vi "NMEA serial.vi"() -> ()   [LabVIEW 2016, in "环境动力监测库.lvlib" / "AIRMAR WeatherCaster.lvlib"]
uses:
  AIRMAR WeatherCaster.lvlib
  NMEA_WIMDA-data.ctl
  NMEA_GPRMC-data.ctl
  NMEA_LatitudeDirection.ctl
  NMEA_LongitudeDirection.ctl
  <vilib>/Utility/miscctls.llb/LVPointTypeDef.ctl
  <vilib>/Instr/_visa.llb/VISA Configure Serial Port (Instr).vi
  <vilib>/ptbypt/NI_PtbyPt.lvlib
  <vilib>/Utility/config.llb/NI_LVConfig.lvlib
panel:
  out "气温":dbl
  out "气压":dbl
  out "风速":dbl
  out "风向":dbl
  out "偏移量/米":dbl format="%#.2f"
  out "纬度":dbl
  out "经度":dbl
  out "时间":timestamp format="%<%H:%M:%S>T"
  out "日期":timestamp format="%<%Y/%m/%d>T"
  out "浮标投放点":cluster{"纬度":dbl, "经度":dbl}
  out "波特率":u32
  out "串口":string
  out "WIMDA signal":bool=TRUE
  in  "重新定标":bool
  in  "移位报警设定值":u32=1000
  out "$GPRMC-message_OUT":T1={"TimeStamp"=timestamp(0 s since 1904-01-01), "Validity"=FALSE, "Latitude"=0.0, "Latitude-Direction"=enum."North", "Longitude"=0.0, "Longitude-Direction"=enum."East", "Speed in knots"=0.0, "True course"=0.0, "Date Stamp"=timestamp(0 s since 1904-01-01), "Magnetic Variation (East/West)"=0.0} {"Magnetic Variation (East/West)" format="%.02f [deg]"; "Date Stamp" format="%<%x>T"; "True course" format="%.02f [deg]"; "Speed in knots" format="%.02f [kts]"; "Longitude" format="%0.4f [long]"; "Latitude" format="%.04f [lat]"; "TimeStamp" format="%<%.2X>T"}
  out "匹配语句":string
  out "$WIMDA-message_OUT":T4
  in  "串口打开":bool
  out "RAW DATA":string
  in  "baud rate (9600)":u32(ring)=4800 caption="波特率" items=["1200"=1200, "2400"=2400, "4800"=4800, "9600"=9600, "38400"=38400, "115200"=115200]
  in  "VISA resource name":refnum<visa-resource-name> caption="串口"
  # "℃"
  # "bars"
  # "m/s"
  # "米"
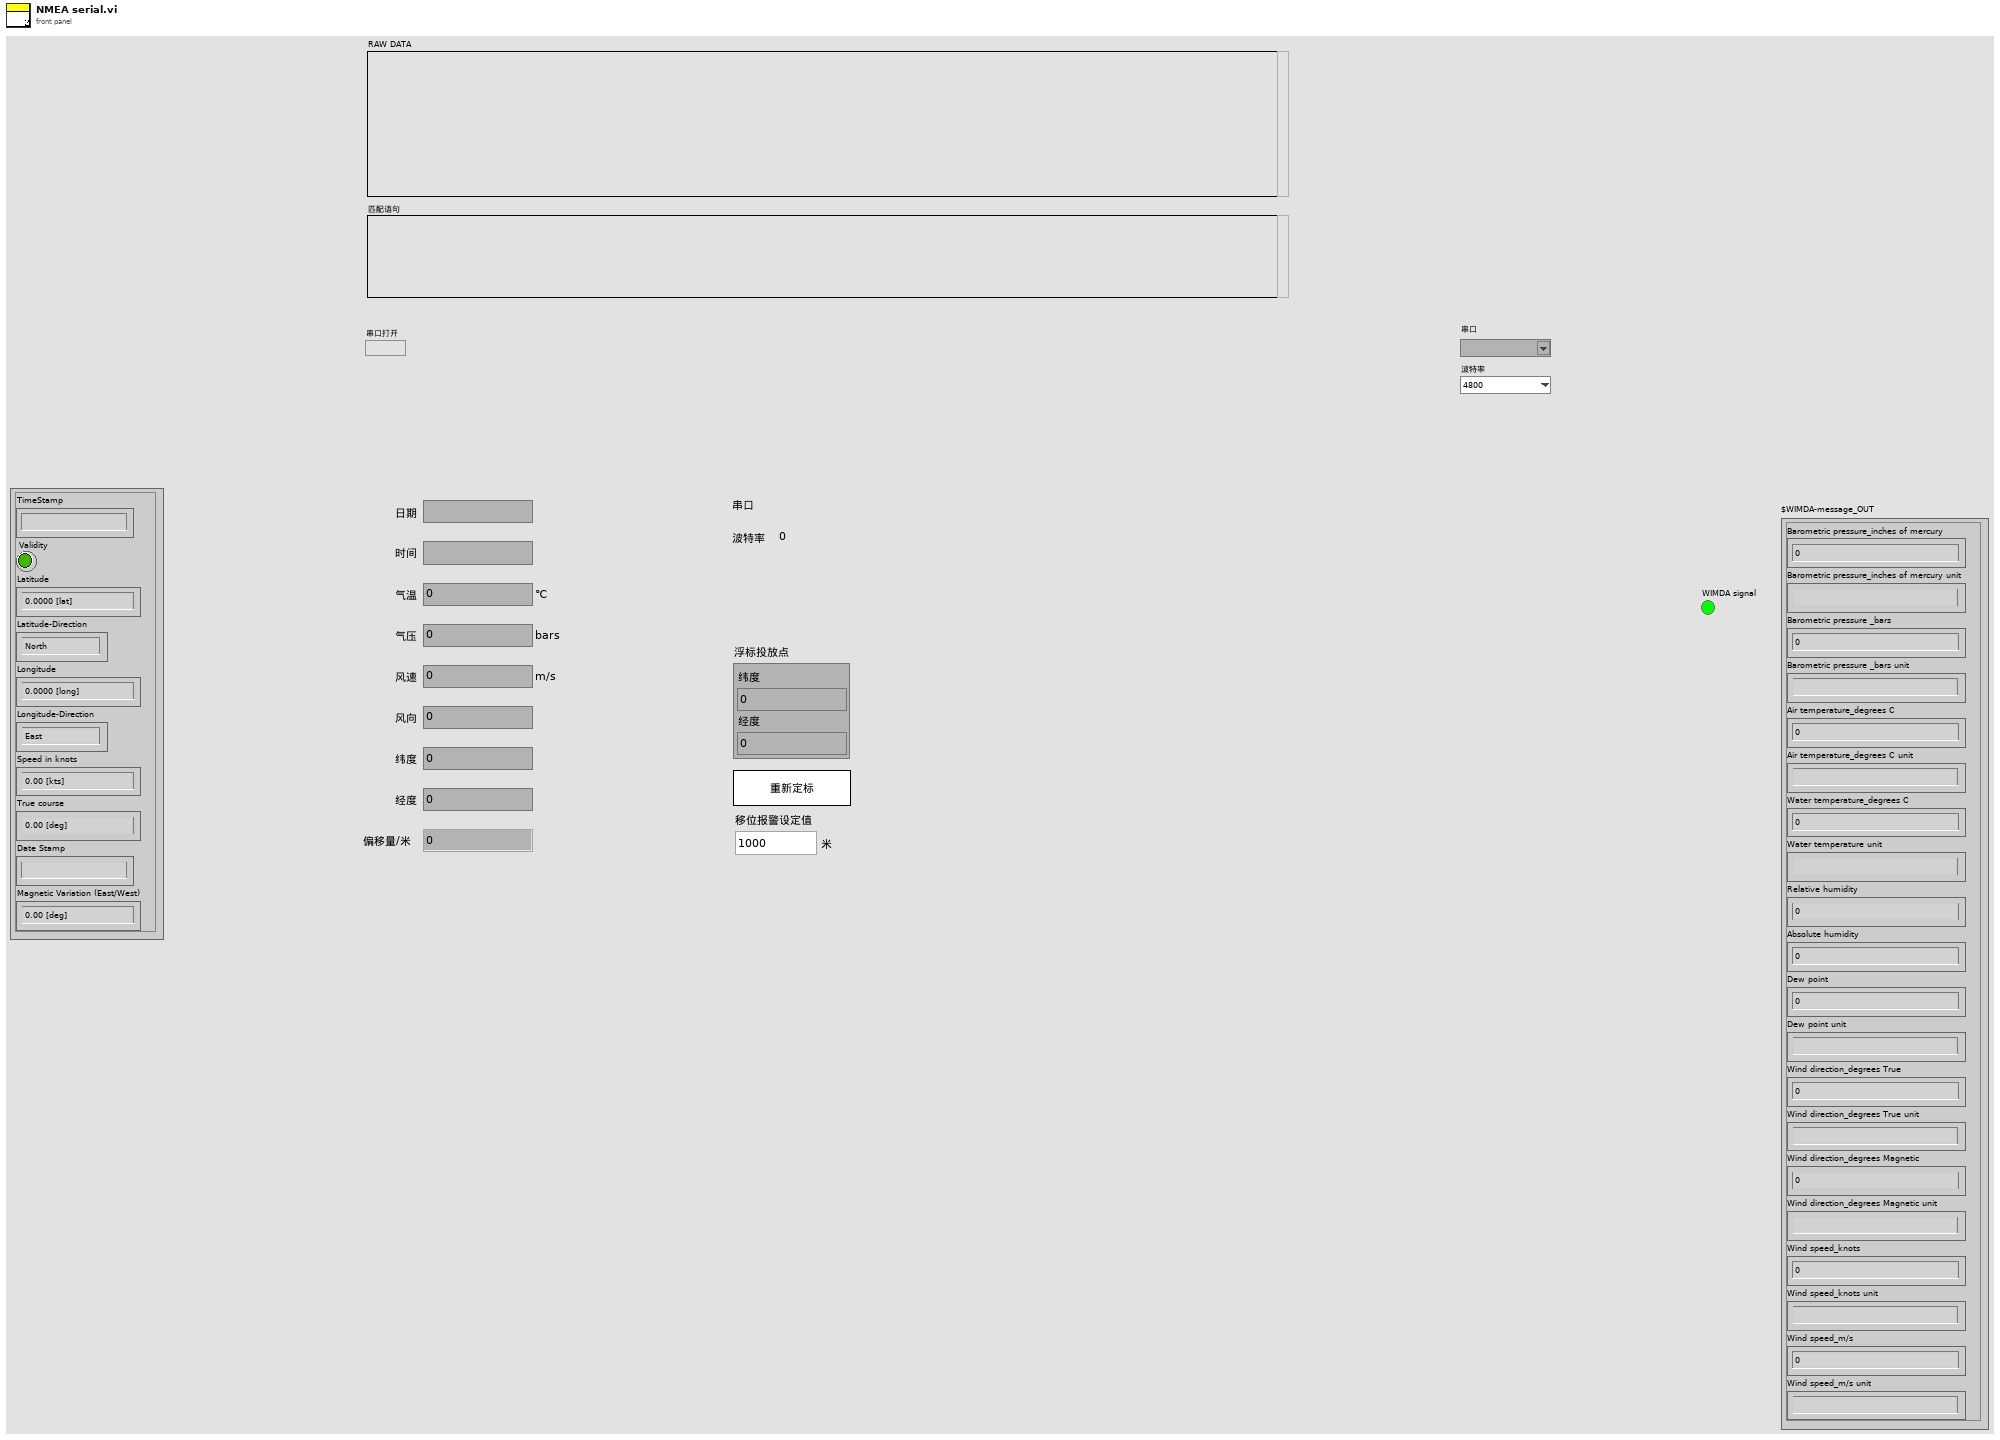
[diagram p1: front panel]
types:
  T1 = typedef "环境动力监测库.lvlib/AIRMAR WeatherCaster.lvlib/NMEA_GPRMC-data.ctl" = cluster{"TimeStamp":timestamp, "Validity":bool, "Latitude":dbl, "Latitude-Direction":T2, "Longitude":dbl, "Longitude-Direction":T3, "Speed in knots":dbl, "True course":dbl, "Date Stamp":timestamp, "Magnetic Variation (East/West)":dbl}
  T2 = typedef "环境动力监测库.lvlib/AIRMAR WeatherCaster.lvlib/NMEA_LatitudeDirection.ctl" = enum16{"", "North", "South"}
  T3 = typedef "环境动力监测库.lvlib/AIRMAR WeatherCaster.lvlib/NMEA_LongitudeDirection.ctl" = enum16{"", "East", "West"}
  T4 = typedef "环境动力监测库.lvlib/AIRMAR WeatherCaster.lvlib/NMEA_WIMDA-data.ctl" = cluster{"Barometric pressure_inches of mercury":dbl, "Barometric pressure_inches of mercury unit":string, "Barometric pressure _bars":dbl, "Barometric pressure _bars unit":string, "Air temperature_degrees C":dbl, "Air temperature_degrees C unit":string, "Water temperature_degrees C":dbl, "Water temperature unit":string, "Relative humidity":dbl, "Absolute humidity":dbl, "Dew point":dbl, "Dew point unit":string, "Wind direction_degrees True":dbl, "Wind direction_degrees True unit":string, "Wind direction_degrees Magnetic":dbl, "Wind direction_degrees Magnetic unit":string, "Wind speed_knots":dbl, "Wind speed_knots unit":string, "Wind speed_m/s":dbl, "Wind speed_m/s unit":string}
  T5 = typedef "LVPointTypeDef.ctl" = cluster{"Horizontal":i16, "Vertical":i16}
  T6 = typedef "LVDateTimeRec.ctl" = cluster{"秒数的小数部分":dbl, "秒":i32, "分":i32, "时":i32, "日":i32, "月":i32, "年":i32, "天数（周）":i32, "天数（年）":i32, "DST":i32}
  T7 = cluster{"漏水监测输出":cluster{"漏水监测告警":bool, "告警内容":string}, "门禁监测输出":cluster{"门禁监测告警":bool, "告警内容":string}, "门禁监测输出2":cluster{"门禁监测告警":bool, "告警内容":string}, "温湿度监测输出":cluster{"温湿度监测告警":bool, "告警内容":string}, "烟雾监测输出":cluster{"烟雾监测告警":bool, "告警内容":string}, "空调监测输出":cluster{"空调监测告警":bool, "告警内容":string}, "自动重合闸输出":cluster{"自动重合闸告警":bool, "告警内容":string}, "红外入侵输出":cluster{"红外入侵告警":bool, "告警内容":string}, "振动输出":cluster{"振动告警":bool, "告警内容":string}, "UPS输出":cluster{"UPS告警":bool, "告警内容":string}, "蓄电池输出":cluster{"蓄电池告警":bool, "告警内容":string}, "蓄电池输出2":cluster{"蓄电池告警":bool, "告警内容":string}, "GPS输出":cluster{"定位告警":bool, "告警内容":string}, "北斗输出":cluster{"定位告警":bool, "告警内容":string}, "气象输出":cluster{"气象告警":bool, "告警内容":string}, "废液输出":cluster{"废液告警":bool, "告警内容":string}, "废液输出2":cluster{"废液告警":bool, "告警内容":string}}
  T8 = cluster{"监测项描述:输出":string, "连接方式":enum16{"串口", "TCP"}, "端口":string, "IP address:":string, "Port:":string, "站号":u64, "传感器型号":string, "波特率":u64, "data bits":u64, "停止位":u16, "奇偶校验":u16}
  T9 = typedef "NI_LVConfig.lvlib/Config Data RefNum.ctl" = refnum<k1>
  T10 = enum8{"Enabled", "Disabled", "Disabled and Grayed Out"}
  T11 = cluster{"传感器":cluster{"红外监测":cluster{"红外监测":bool, "红外入侵监测":bool}, "振动监测":cluster{"振动监测":bool, "振动监测 2":bool}, "烟雾监测":cluster{"烟雾监测":bool, "烟雾监测 2":bool}, "门禁监测":cluster{"门禁监测":bool, "门禁开关监测":bool}, "门禁2监测":cluster{"门禁监测2":bool, "门禁开关监测2":bool}, "水浸监测":cluster{"水浸监测":bool, "漏水详情":bool}, "废液监测":cluster{"废液监测":bool, "废液详情":bool}, "废液监测2":cluster{"废液监测2":bool, "废液2详情":bool}}, "气象仪":cluster{"气温: ":sgl, "气压: ":sgl, "风速:":sgl, "风向:":sgl, "气象仪经度: ":sgl, "气象仪纬度: ":sgl, "详情  ":bool}}
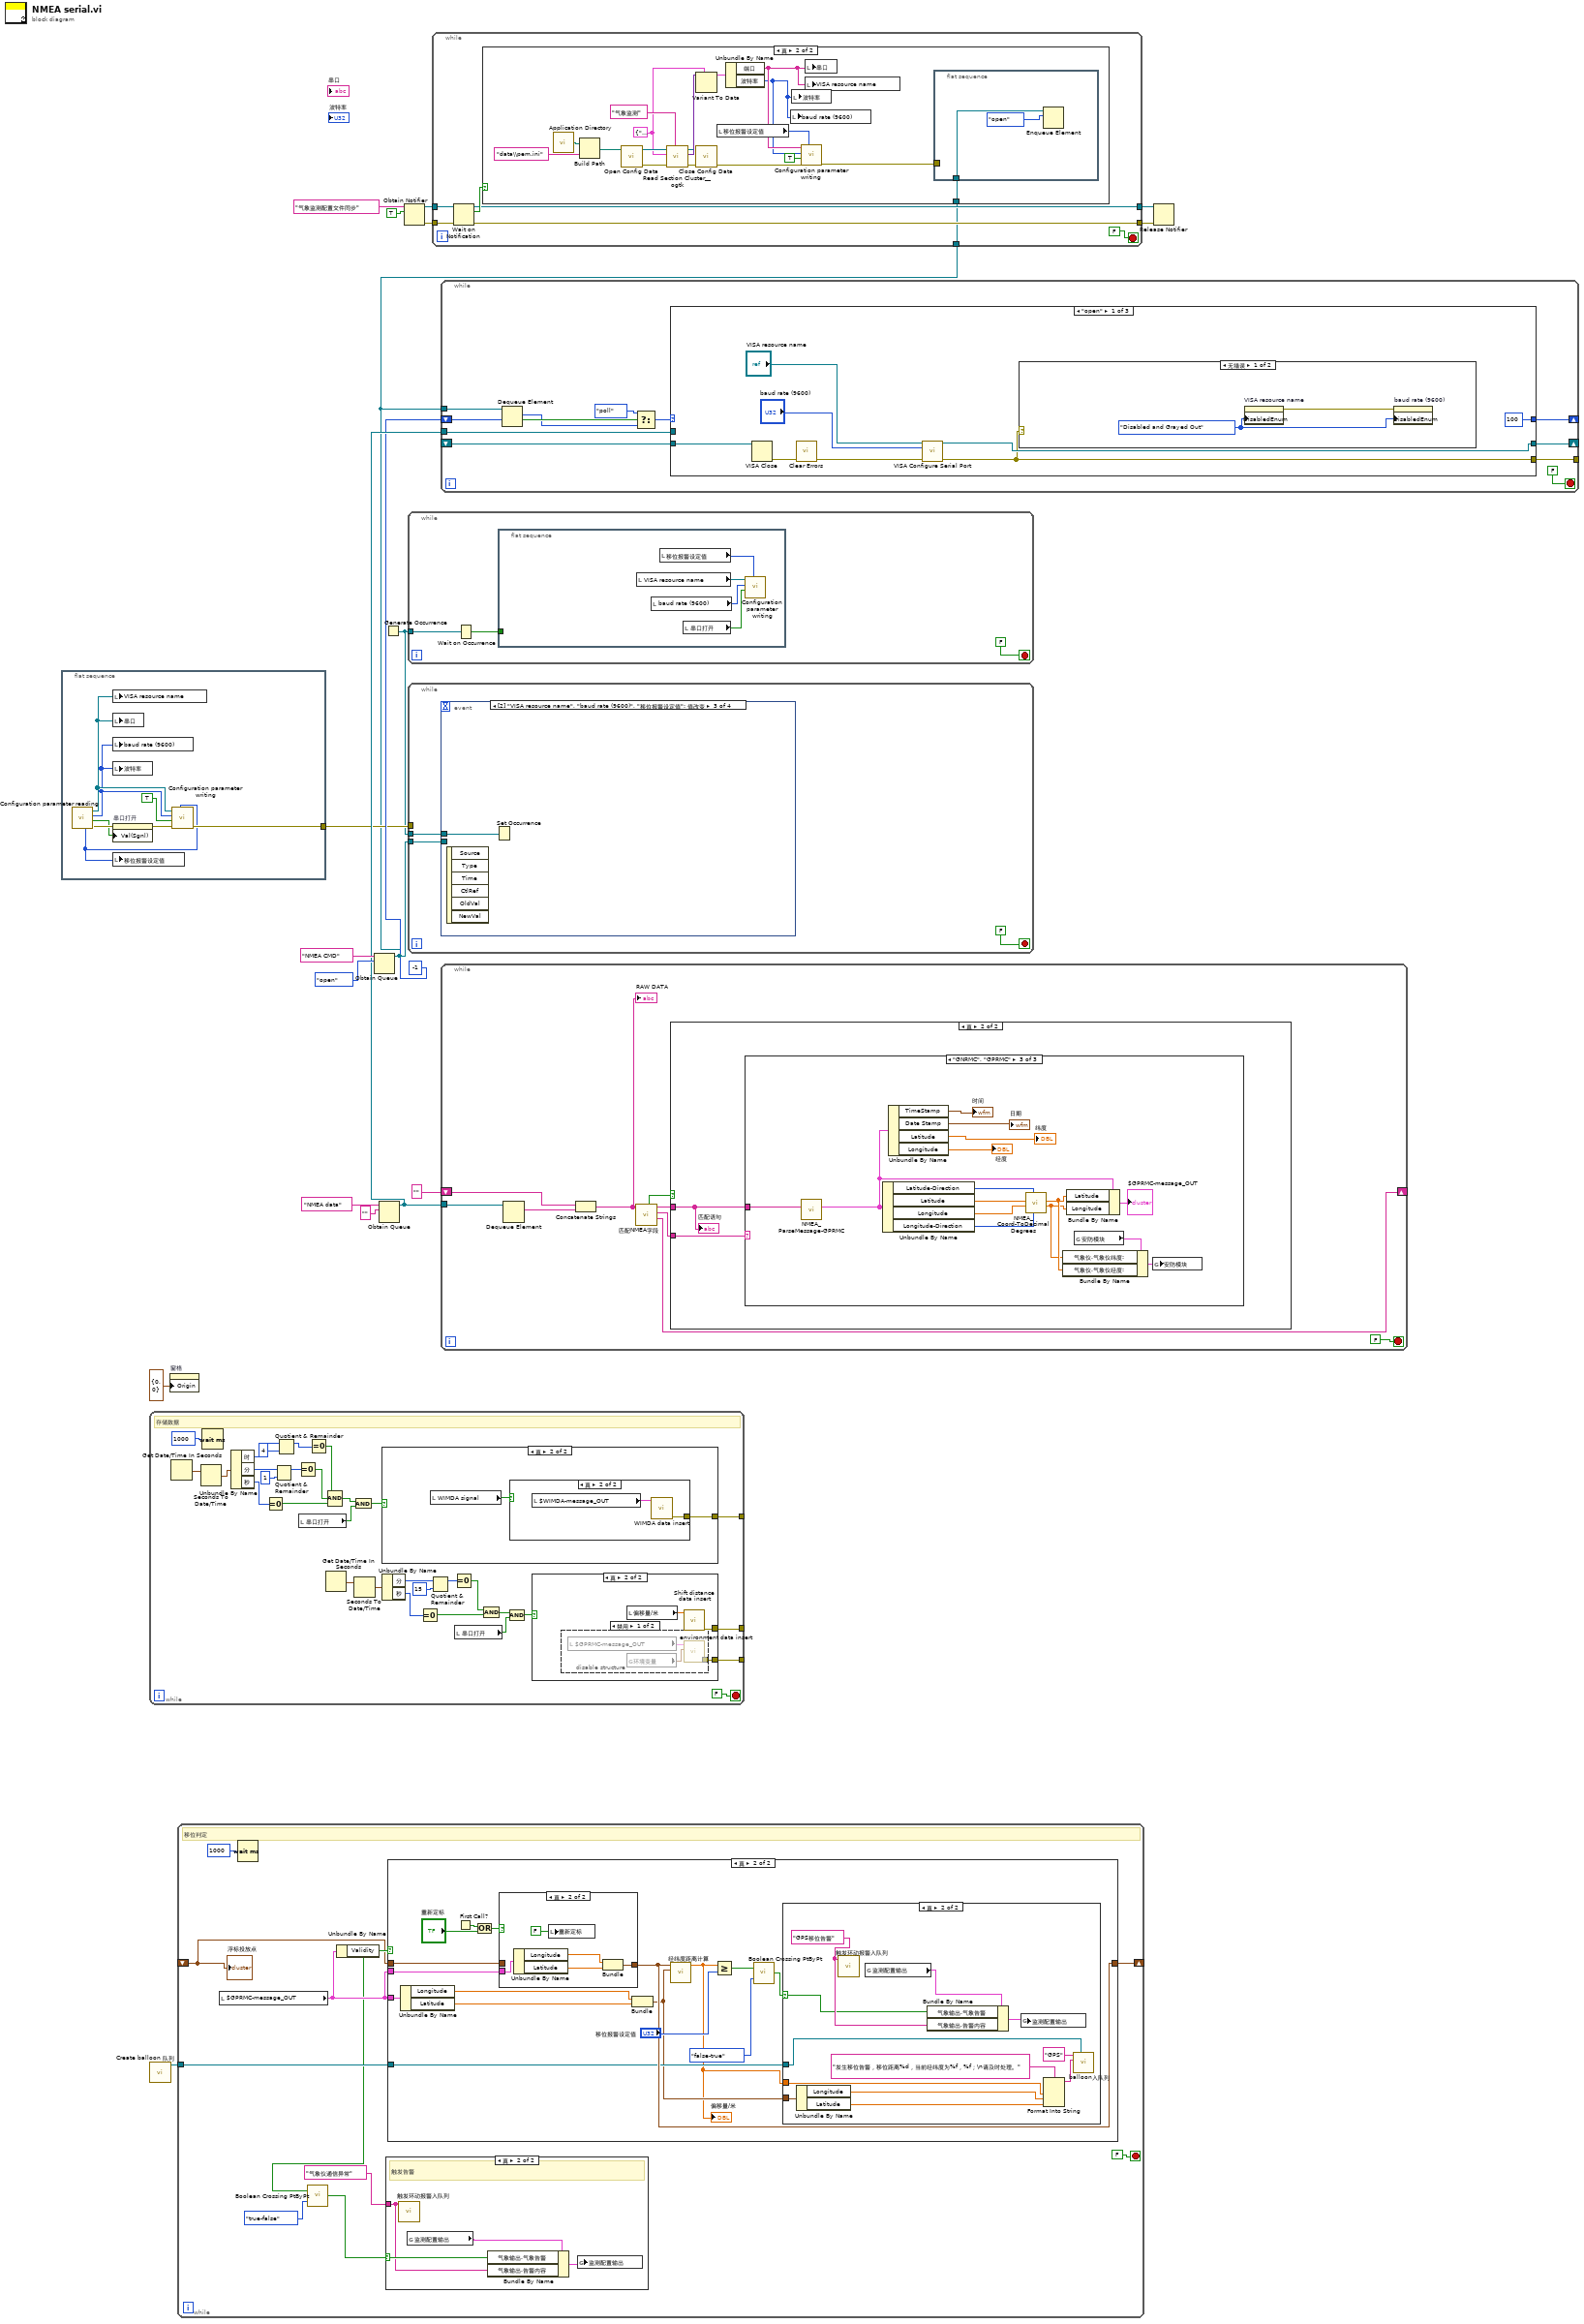
[diagram p0: block diagram]
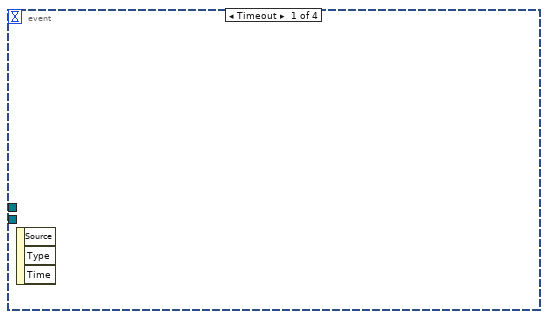
[diagram p11: hidden frame]
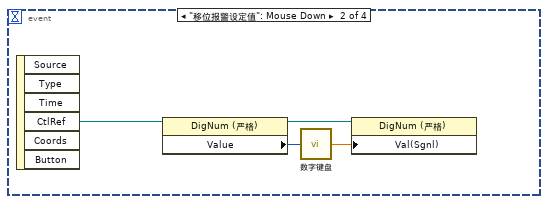
[diagram p12: hidden frame]
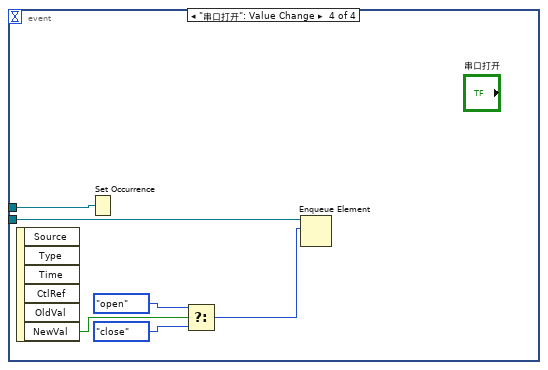
[diagram p13: hidden frame]
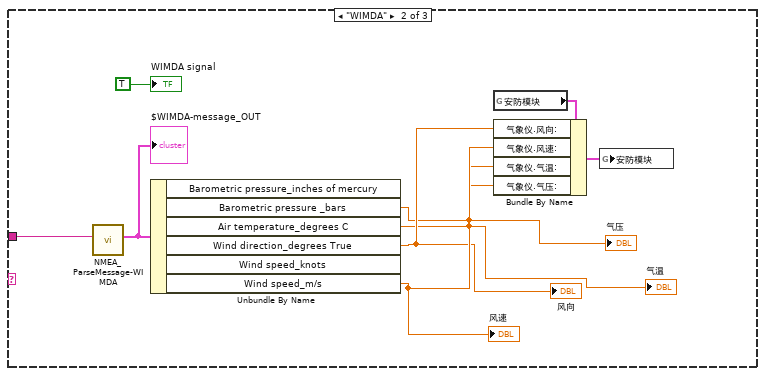
[diagram p16: hidden frame]
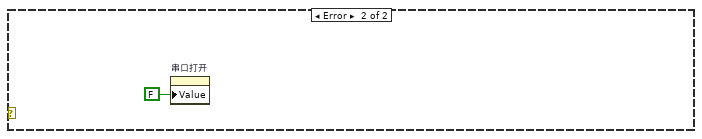
[diagram p17: hidden frame]
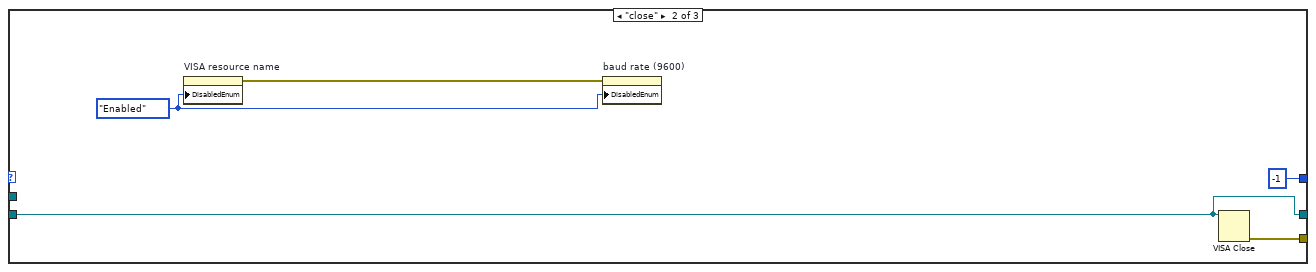
[diagram p18: hidden frame]
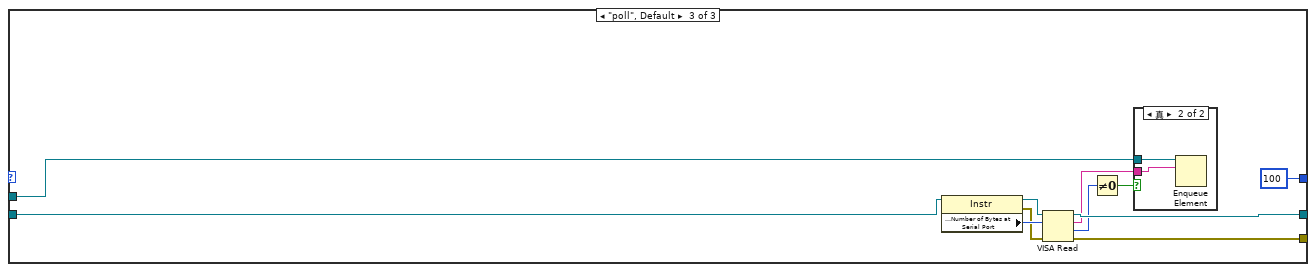
[diagram p19: hidden frame]
diagram:
  n1 = flat-sequence {
    tunnel: [w20] -> w10
    frame #0 {
      n2 = call "Configuration parameter reading.vi"() -> ("error out"=w26:errorcluster, "enable"=w25:bool, "baud rate (9600)"=w23:u32, "VISA resource name"=w24:refnum<visa-resource-name>, "Shift distance"=w19:u32)  [unwired: 7 in]
      n3 = local write "VISA resource name"(w24) -> ()
      n4 = local write "串口"(w24) -> ()
      n5 = local write "baud rate (9600)"(w23) -> ()
      n6 = local write "波特率"(w23) -> ()
      n7 = property on="串口打开" class="Bool (严格)"(error in=w26, "Val(Sgnl)"=w25) -> (error out=w21:errorcluster)  [unwired: 1 in, 1 out]
      n8 = local write "移位报警设定值"(w19) -> ()
      n9 = call "Configuration parameter writing.vi"("Shift distance"=w19, "error in (no error)"=w21, "enable"=TRUE, "baud rate (9600)"=w23, "VISA resource name"=w24) -> ("error out"=w20:errorcluster)  [unwired: 6 in]
    }
  }
  n10 = while {
    tunnel: [w35] -> _
    tunnel: [w34] -> _
    tunnel: [w33] -> _
    stop <- FALSE stop-if-true
    # "存储数据"
    n11 = Get Date/Time In Seconds() -> (seconds since 1Jan1904=w48:timestamp)
    n12 = Seconds To Date/Time(time stamp (now)=w48) -> (date time rec=w56:T6)  [unwired: 1 in]
    n13 = Wait (ms)(milliseconds to wait=u32 1000 ("等待时间（毫秒）")) -> ()  [unwired: 1 out]
    n14 = Unbundle By Name(w56) -> ("时"=w30:i32, "分"=w55:i32, "秒"=w52:i32)
    n15 = Equal To 0?(x=w52) -> (x = 0?=w50:bool)
    n16 = Quotient & Remainder(x=w55, y=1) -> (x-y*floor(x/y)=w53:i32)  [unwired: 1 out]
    n17 = Quotient & Remainder(x=w30, y=4) -> (x-y*floor(x/y)=w28:i32)  [unwired: 1 out]
    n18 = Equal To 0?(x=w53) -> (x = 0?=w51:bool)
    n19 = local read "串口打开"() -> (w45:bool)
    n20 = Equal To 0?(x=w28) -> (x = 0?=w27:bool)
    n21 = Get Date/Time In Seconds() -> (seconds since 1Jan1904=w44:timestamp)
    n22 = Compound Arithmetic op=AND ("复合运算")(w27, w51, w50) -> (w49:bool)
    n23 = And(x=w49, y=w45) -> (x .and. y?=w46:bool)
    n24 = Seconds To Date/Time(time stamp (now)=w44) -> (date time rec=w37:T6)  [unwired: 1 in]
    n25 = case shown="真" w46 {
      tunnel: [_ w65] -> w34
      frame False {
      }
      frame True {
        n26 = local read "WIMDA signal"() -> (w64:bool)
        n27 = case shown="真" w64 {
          tunnel: [_ w66] -> w65
          frame False {
          }
          frame True {
            n28 = local read "$WIMDA-message_OUT"() -> (w67:T4)
            n29 = call "WIMDA data insert.vi"("WIMDA-data"=w67) -> ("error out"=w66:errorcluster)  [unwired: 10 in]
          }
        }
      }
    }
    n30 = Unbundle By Name(w37) -> ("分"=w38:i32, "秒"=w41:i32)
    n31 = Equal To 0?(x=w41) -> (x = 0?=w43:bool)
    n32 = Quotient & Remainder(x=w38, y=15) -> (x-y*floor(x/y)=w40:i32)  [unwired: 1 out]
    n33 = Equal To 0?(x=w40) -> (x = 0?=w42:bool)
    n34 = local read "串口打开"() -> (w32:bool)
    n35 = And(x=w42, y=w43) -> (x .and. y?=w31:bool)
    n36 = Compound Arithmetic op=AND ("复合运算")(w31, w32) -> (w36:bool)
    n37 = case shown="真" w36 {
      tunnel: [_ w60] -> w35
      tunnel: [_ w59] -> w33
      frame False {
      }
      frame True {
        n38 = disable-structure shown="禁用" {
          disable-tunnel: [w63 _] -> w60
          frame Disabled {
            n39 = local read "$GPRMC-message_OUT"() -> (w62:T1)
            n40 = global read "气象全局变量.vi" "环境变量"() -> (w61:cluster{"电压":dbl, "室温":dbl, "湿度":dbl})
            n41 = call "environment data insert.vi"("环境变量"=w61, "$GPRMC-message_OUT"=w62) -> ("error out"=w63:errorcluster)  [unwired: 9 in]
          }
          frame Enabled {
          }
        }
        n42 = local read "偏移量/米"() -> (w58:dbl)
        n43 = call "Shift distance data insert.vi"("移位距离"=w58) -> ("error out"=w59:errorcluster)  [unwired: 10 in]
      }
    }
  }
  n44 = call "Create balloon 队列.vi"() -> ("队列输出"=w8:refnum<queue>)  [unwired: 11 in]
  n45 = property on="窗格" class="Pane"("Origin"=T5 {"Horizontal"=0, "Vertical"=0} ("原点")) -> ()  [unwired: 2 in, 2 out]
  n46 = while {
    shift-right: [w77] -> _
    shift-left: _ -> [w68]
    tunnel: w8 -> [w73]
    stop <- FALSE stop-if-true
    # "移位判定"
    n47 = local read "$GPRMC-message_OUT"() -> (w75:T1)
    n48 = Wait (ms)(milliseconds to wait=u32 1000 ("等待时间（毫秒）")) -> ()  [unwired: 1 out]
    n49 = Unbundle By Name(w75) -> ("Validity"=w69:bool)
    n50 = call <vilib>:"Boolean Crossing PtByPt.vi"("direction"=enum16{"either", "false-true", "true-false"}."true-false", "input"=w69) -> ("crossing"=w71:bool)  [unwired: 1 in]
    n51 = case shown="真" w71 {
      selector: w71 -> [_ w81]
      tunnel: "气象仪通信异常" ("设备") -> [_ w80]
      frame False {
      }
      frame True {
        # "触发告警"
        n52 = call "触发环动报警入队列.vi"("报警内容"=w80) -> ()  [unwired: 11 in]
        n53 = global read "内部交互全局变量.vi" "监测配置输出"() -> (w79:T7)
        n54 = Bundle By Name(cluster=w79, "气象输出.气象告警"=w81, "气象输出.告警内容"=w80) -> (w78:T7)
        n55 = global write "内部交互全局变量.vi" "监测配置输出"(w78) -> ()
      }
    }
    n56 = case shown="真" w69 {
      tunnel: [w82 w96] -> w77
      tunnel: w68 -> [w82 w95]
      tunnel: w75 -> [_ w94]
      tunnel: w75 -> [_ w93]
      tunnel: w73 -> [_ w89]
      frame False {
      }
      frame True {
        n57 = Unbundle By Name(w93) -> ("Longitude"=w98:dbl, "Latitude"=w97:dbl)
        n58 = First Call?() -> (First Call?: T/F=w92:bool)
        n59 = Or(x=w92, y="重新定标") -> (x .or. y?=w91:bool)
        n60 = case shown="真" w91 {
          tunnel: [w111 w114] -> w96
          tunnel: w95 -> [w111 _]
          tunnel: w94 -> [_ w113]
          frame False {
          }
          frame True {
            n61 = Unbundle By Name(w113) -> ("Longitude"=w115:dbl, "Latitude"=w116:dbl)
            n62 = local write "重新定标"(FALSE ("重新定标")) -> ()
            n63 = Bundle("Longitude"=w115, "Latitude"=w116) -> (w114:cluster{"Longitude":dbl, "Latitude":dbl})  [unwired: 1 in]
          }
        }
        n64 = Bundle("Longitude"=w98, "Latitude"=w97) -> (w84:cluster{"Longitude":dbl, "Latitude":dbl})  [unwired: 1 in]
        n65 = call "经纬度距离计算.vi"("结束位置"=w84, "起始位置"=w96) -> ("距离"=w83:dbl)  [unwired: 9 in]
        "偏移量/米" <- w83
        n66 = Greater Or Equal?(x=w83, y="移位报警设定值") -> (x >= y?=w87:bool)
        n67 = call <vilib>:"Boolean Crossing PtByPt.vi"("direction"=enum16{"either", "false-true", "true-false"}."false-true", "input"=w87) -> ("crossing"=w85:bool)  [unwired: 1 in]
        n68 = case shown="真" w85 {
          selector: w85 -> [_ w101]
          tunnel: w89 -> [_ w110]
          tunnel: w83 -> [_ w106]
          tunnel: w84 -> [_ w105]
          frame False {
          }
          frame True {
            w102 = "GPS移位告警" ("参数名称")
            n69 = Unbundle By Name(w105) -> ("Longitude"=w104:dbl, "Latitude"=w103:dbl)
            n70 = call "触发环动报警入队列.vi"("报警内容"=w102) -> ()  [unwired: 11 in]
            n71 = global read "内部交互全局变量.vi" "监测配置输出"() -> (w100:T7)
            n72 = Bundle By Name(cluster=w100, "气象输出.气象告警"=w101, "气象输出.告警内容"=w102) -> (w99:T7)
            n73 = global write "内部交互全局变量.vi" "监测配置输出"(w99) -> ()
            n74 = Format Into String(format string="发生移位告警，移位距离%d，当前经纬度为%f，%f；\n请及时处理。" ("格式字符串"), w106, w104, w103) -> (resulting string=w107:string)  [unwired: 2 in, 1 out]
            n75 = call "balloon入队列.vi"("队列"=w110, "故障信息"=w107, "参数名称"="GPS") -> ()  [unwired: 8 in, 1 out]
          }
        }
      }
    }
    "浮标投放点" <- w68
  }
  n76 = Obtain Queue(name (unnamed)="NMEA CMD" ("名称（未命名）"), element data type=enum16{"open", "close", "poll"}."open" ("枚举")) -> (queue out=w1:refnum<queue>)  [unwired: 3 in, 2 out]
  n77 = Obtain Queue(name (unnamed)="NMEA data" ("名称（未命名）"), element data type="") -> (queue out=w14:refnum<queue>)  [unwired: 3 in, 2 out]
  n78 = Generate Occurrence() -> (w9:refnum<k4>)
  n79 = Obtain Notifier(name (unnamed)="气象监测配置文件同步" ("名称（未命名）"), notification data type=TRUE) -> (notifier out=w5:refnum<notifier>, error out=w4:errorcluster)  [unwired: 2 in, 1 out]
  n80 = while {
    tunnel: w9 -> [w118]
    stop <- FALSE stop-if-true
    n81 = Wait on Occurrence(2:w118) -> (0:w117:bool)  [unwired: 2 in]
    n82 = flat-sequence {
      tunnel: w117 -> [_]
      frame #0 {
        n83 = local read "VISA resource name"() -> (w123:refnum<visa-resource-name>)
        n84 = local read "baud rate (9600)"() -> (w122:u32)
        n85 = local read "移位报警设定值"() -> (w120:u32)
        n86 = local read "串口打开"() -> (w121:bool)
        n87 = call "Configuration parameter writing.vi"("Shift distance"=w120, "enable"=w121, "baud rate (9600)"=w122, "VISA resource name"=w123) -> ()  [unwired: 7 in, 1 out]
      }
    }
  }
  n88 = while {
    tunnel: w1 -> [w125]
    tunnel: w10 -> [_]
    tunnel: w9 -> [w124]
    stop <- FALSE stop-if-true
    n89 = event shown="[2] \"VISA resource name\", \"baud rate (9600)\", \"移位报警设定值\": 值改变" {
      selector: _ -> [_ _ _ _]
      dyn-events: _ -> [_ _ _ _]
      timeout: _ -> [_ _ _ _]
      tunnel: w125 -> [_ _ _ w137]
      tunnel: w124 -> [_ _ w131 w132]
      event Timeout {
        n90 = event-data() -> ()  [unwired: 1 in, 3 out]
      }
      event "移位报警设定值": Mouse Down {
        n91 = event-data() -> ("CtlRef"=w130:refnum<vi>)  [unwired: 1 in, 5 out]
        n92 = property class="DigNum (严格)"(reference=w130) -> (reference out=w129:refnum<vi>, "Value"=w128:u32)  [unwired: 1 in, 1 out]
        n93 = call "数字键盘.vi"("OldNumber"=w128) -> ("NewNumber"=w127:sgl)
        n94 = property class="DigNum (严格)"(reference=w129, "Val(Sgnl)"=w127) -> ()  [unwired: 1 in, 2 out]
      }
      event "VISA resource name", "baud rate (9600)", "移位报警设定值": Value Change {
        n95 = event-data() -> ()  [unwired: 1 in, 6 out]
        n96 = Set Occurrence(w131) -> ()
      }
      event "串口打开": Value Change {
        n97 = event-data() -> ("NewVal"=w136:bool)  [unwired: 1 in, 5 out]
        n98 = Set Occurrence(w132) -> ()
        n99 = Select(t=enum16{"open", "close", "poll"}."open" ("元素"), s=w136, f=enum16{"open", "close", "poll"}."close") -> (s? t:f=w134:enum16{"open", "close", "poll"})
        n100 = Enqueue Element(queue=w137, element=w134) -> ()  [unwired: 2 in, 3 out]
      }
    }
  }
  n101 = while {
    tunnel: w5 -> [w144]
    tunnel: w4 -> [w143]
    tunnel: [w140] -> w3
    tunnel: [w139] -> w2
    tunnel: w1 -> [w138]
    stop <- FALSE stop-if-true
    n102 = Wait on Notification(notifier=w144, error in (no error)=w143) -> (notifier out=w140:refnum<notifier>, notification=w142:bool, error out=w139:errorcluster)  [unwired: 2 in, 1 out]
    n103 = case shown="真" w142 {
      tunnel: w138 -> [_ w151]
      frame False {
      }
      frame True {
        w152 = T8 {"监测项描述:输出"="", "连接方式"=enum."串口", "端口"="", "IP address:"="", "Port:"="", "站号"=19200, "传感器型号"="", "波特率"=19200, "data bits"=8, "停止位"=10, "奇偶校验"=0} ("输入簇")
        n104 = call <vilib>:"Application Directory.vi"() -> ("Application Directory"=w156:path)
        n105 = Build Path(base path=w156, name or relative path="data\\pem.ini" ("名称或相对路径")) -> (appended path=w155:path)
        n106 = call <vilib>:"Open Config Data.vi"("configuration file path"=w155) -> ("error out"=w154:errorcluster, "refnum"=w153:T9)  [unwired: 8 in, 1 out]
        n107 = call <userlib>:"Read Section Cluster__ogtk.vi"("section (optional)"="气象监测", "error in (no error)"=w154, "Section Formatted Cluster Type"=w152, "refnum"=w153) -> ("error out"=w160:errorcluster, "Section Formatted Cluster"=w161:variant, "dup refnum"=w159:T9)  [unwired: 3 in, 2 out]
        n108 = Variant To Data(type=w152, Variant=w161) -> (data=w162:T8)  [unwired: 1 in, 1 out]
        n109 = call <vilib>:"Close Config Data.vi"("error in (no error)"=w160, "refnum"=w159) -> ("error out"=w150:errorcluster)  [unwired: 8 in, 1 out]
        n110 = local read "移位报警设定值"() -> (w145:u32)
        n111 = Unbundle By Name(w162) -> ("端口"=w149:string, "波特率"=w148:u64)
        n112 = local write "baud rate (9600)"(w148) -> ()
        n113 = local write "波特率"(w148) -> ()
        n114 = call "Configuration parameter writing.vi"("Shift distance"=w145, "error in (no error)"=w150, "enable"=TRUE, "baud rate (9600)"=w148, "VISA resource name"=w149) -> ("error out"=w146:errorcluster)  [unwired: 6 in]
        n115 = local write "串口"(w149) -> ()
        n116 = local write "VISA resource name"(w149) -> ()
        n117 = flat-sequence {
          tunnel: w151 -> [w164]
          tunnel: w146 -> [_]
          frame #0 {
            n118 = Enqueue Element(queue=w164, element=enum16{"open", "close", "poll"}."open" ("枚举")) -> ()  [unwired: 2 in, 3 out]
          }
        }
      }
    }
  }
  n119 = while {
    shift-right: [w176] -> _
    shift-left: _ -> [w175]
    tunnel: w1 -> [w174]
    tunnel: [w173] -> _
    tunnel: w14 -> [w172]
    shift-right: [w165] -> _
    shift-left: -1 ("超时毫秒(-1)") -> [w166]
    stop <- FALSE stop-if-true
    n120 = Dequeue Element(queue=w174, timeout in ms (-1)=w166) -> (element=w168:enum16{"open", "close", "poll"}, timed out?=w170:bool)  [unwired: 1 in, 2 out]
    n121 = Select(t=enum16{"open", "close", "poll"}."poll" ("枚举"), s=w170, f=w168) -> (s? t:f=w167:enum16{"open", "close", "poll"})
    n122 = case shown="\"open\"" w167 {
      tunnel: [w182 w192 w203] -> w176
      tunnel: w175 -> [w181 w192 w201]
      tunnel: [w177 w191 w202] -> w173
      tunnel: w172 -> [_ _ w198]
      tunnel: [100 ("超时毫秒(-1)") -1 ("超时毫秒(-1)") 100 ("超时毫秒(-1)")] -> w165
      frame "open" {
        n123 = VISA Close(VISA resource name=w181) -> (error out=w180:errorcluster)  [unwired: 1 in]
        n124 = call <vilib>:"Clear Errors.vi"("error in (no error)"=w180) -> ("error out"=w179:errorcluster)  [unwired: 5 in, 1 out]
        n125 = call-poly "VISA Configure Serial Port"("VISA resource name"="VISA resource name", "baud rate (9600)"="baud rate (9600)", "error in (no error)"=w179) -> ("VISA resource name out"=w182:refnum<visa-resource-name>, "error out"=w177:errorcluster)  [unwired: 11 in]
        n126 = case shown="无错误" w177 {
          frame No Error {
            w186 = T10."Disabled and Grayed Out" ("禁用")
            n127 = property on="VISA resource name" class="VISAName"("DisabledEnum"=w186) -> (error out=w185:errorcluster)  [unwired: 2 in, 1 out]
            n128 = property on="baud rate (9600)" class="Ring (严格)"(error in=w185, "DisabledEnum"=w186) -> ()  [unwired: 1 in, 2 out]
          }
          frame Error {
            n129 = property on="串口打开" class="Bool (严格)"("Value"=FALSE ("串口打开")) -> ()  [unwired: 2 in, 2 out]
          }
        }
      }
      frame "close" {
        w188 = T10."Enabled" ("禁用")
        n130 = property on="VISA resource name" class="VISAName"("DisabledEnum"=w188) -> (error out=w189:errorcluster)  [unwired: 2 in, 1 out]
        n131 = property on="baud rate (9600)" class="Ring (严格)"(error in=w189, "DisabledEnum"=w188) -> ()  [unwired: 1 in, 2 out]
        n132 = VISA Close(VISA resource name=w192) -> (error out=w191:errorcluster)  [unwired: 1 in]
      }
      frame "poll", Default {
        n133 = property class="Instr"(reference=w201) -> (reference out=w200:refnum<visa-resource-name>, error out=w194:errorcluster, "Serial Settings:Number of Bytes at Serial Port"=w199:u32)  [unwired: 1 in]
        n134 = VISA Read(VISA resource name=w200, byte count=w199, error in (no error)=w194) -> (VISA resource name out=w203:refnum<visa-resource-name>, read buffer=w197:string, return count=w196:u32, error out=w202:errorcluster)
        n135 = Not Equal To 0?(x=w196) -> (x != 0?=w195:bool)
        n136 = case shown="真" w195 {
          tunnel: w198 -> [_ w205]
          tunnel: w197 -> [_ w204]
          frame False {
          }
          frame True {
            n137 = Enqueue Element(queue=w205, element=w204) -> ()  [unwired: 2 in, 3 out]
          }
        }
      }
    }
  }
  n138 = while {
    tunnel: w14 -> [w214]
    shift-right: [w207] -> _
    shift-left: "" -> [w212]
    stop <- FALSE stop-if-true
    n139 = Dequeue Element(queue=w214) -> (element=w213:string)  [unwired: 2 in, 3 out]
    n140 = Concatenate Strings(w212, w213) -> (w210:string)
    "RAW DATA" <- w210
    n141 = call "匹配NMEA字段.vi"("输入字符串"=w210) -> ("未匹配语句"=w207:string, "NMEA语句"=w206:string, "匹配语句"=w209:string, "匹配"=w208:bool)  [unwired: 7 in]
    n142 = case shown="真" w208 {
      tunnel: w209 -> [_ w216]
      tunnel: w206 -> [_ w215]
      frame False {
      }
      frame True {
        n143 = case shown="\"GNRMC\", \"GPRMC\"" w215 {
          tunnel: w216 -> [_ w225 w240]
          frame "假", Default {
          }
          frame "WIMDA" {
            n144 = call "NMEA_ParseMessage-WIMDA.vi"("$WIMDA-message_IN"=w225) -> ("$WIMDA-message_OUT"=w224:T4)  [unwired: 9 in, 1 out]
            "$WIMDA-message_OUT" <- w224
            n145 = Unbundle By Name(w224) -> ("Barometric pressure _bars"=w218:dbl, "Air temperature_degrees C"=w217:dbl, "Wind direction_degrees True"=w219:dbl, "Wind speed_m/s"=w220:dbl)  [unwired: 2 out]
            "风速" <- w220
            "风向" <- w219
            "气压" <- w218
            "气温" <- w217
            n146 = global read "内部交互全局变量.vi" "安防模块"() -> (w221:T11)
            n147 = Bundle By Name(cluster=w221, "气象仪.风向:"=w219, "气象仪.风速:"=w220, "气象仪.气温:"=w217, "气象仪.气压:"=w218) -> (w222:T11)
            n148 = global write "内部交互全局变量.vi" "安防模块"(w222) -> ()
            "WIMDA signal" <- TRUE ("WIMDA")
          }
          frame "GNRMC", "GPRMC" {
            n149 = call "NMEA_ParseMessage-GPRMC.vi"("$GPRMC-message_IN"=w240) -> ("$GPRMC-message_OUT"=w230:T1)  [unwired: 9 in, 1 out]
            n150 = Unbundle By Name(w230) -> ("Latitude-Direction"=w236:T2, "Latitude"=w239:dbl, "Longitude"=w238:dbl, "Longitude-Direction"=w237:T3)
            n151 = Unbundle By Name(w230) -> ("TimeStamp"=→"时间":timestamp, "Date Stamp"=→"日期":timestamp, "Latitude"=→"纬度":dbl, "Longitude"=→"经度":dbl)
            n152 = call "NMEA_Coord-ToDecimalDegrees.vi"("Longitude-Direction"=w237, "Latitude-Direction"=w236, "Longitude"=w238, "Latitude"=w239) -> ("Longitude"=w231:dbl, "Latitude"=w232:dbl)  [unwired: 6 in]
            n153 = Bundle By Name(cluster=w230, "Latitude"=w232, "Longitude"=w231) -> (→"$GPRMC-message_OUT":T1)
            n154 = global read "内部交互全局变量.vi" "安防模块"() -> (w233:T11)
            n155 = Bundle By Name(cluster=w233, "气象仪.气象仪纬度:"=w231, "气象仪.气象仪经度:"=w232) -> (w234:T11)
            n156 = global write "内部交互全局变量.vi" "安防模块"(w234) -> ()
          }
        }
        "匹配语句" <- w216
      }
    }
  }
  n157 = Release Notifier(notifier=w3, error in (no error)=w2) -> ()  [unwired: 1 in, 3 out]
